vi "test Add Find Remove APU.vi"(8 "error in (no error)":errorcluster, 11 "TestCase in":refnum<class "Scripting API Test Case.lvclass">) -> (0 "error out":errorcluster, 3 "TestCase out":refnum<class "Scripting API Test Case.lvclass">)   [LabVIEW 2019, in "Scripting API Test Case.lvclass"]
uses:
  Scripting API Test Case.lvclass
  Scripting API/Custom Device/Engine Simulation Toolkit Custom Device Settings.ctl
  Scripting API/Bitfile/Bitfile.ctl
  Scripting API/APU/APU Settings.ctl
  Scripting API Test Case.lvclass/Scripting API Test Case.ctl
  <userlib>/_OpenG.lib/file/file.llb/Append Path to Root if Relative - Scalar__ogtk.vi
  <vilib>/addons/_JKI Toolkits/VI Tester/TestCase.llb/TestCase.lvclass
  Scripting API/Engine Simulation Toolkit Scripting API.lvlib
  niveristand-custom-device-testing-tools/VeriStandTestUtilities/VeriStandTestUtilities.lvlib
  C:/Program Files (x86)/National Instruments/LabVIEW 2019/vi.lib/addons/_JKI Toolkits/VI Tester/TestCase.llb/TestCase.lvclass
panel:
  in  "Save?":bool
  out "Output Filename":string
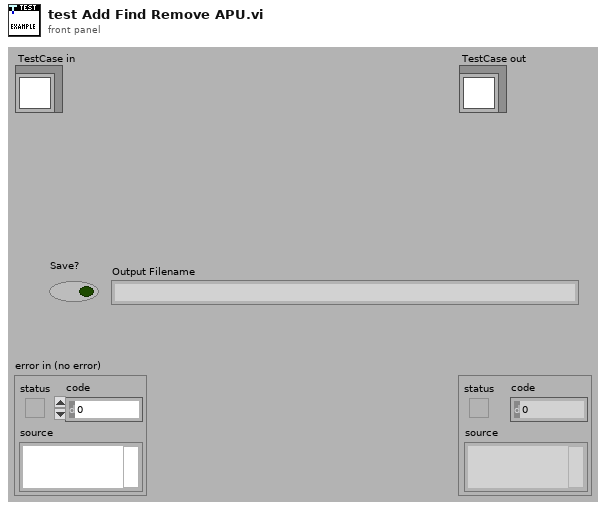
[diagram p1: front panel]
types:
  T1 = typedef "Engine Simulation Toolkit Scripting API.lvlib/APU Settings.ctl" = cluster{"Name":string, "Start angle (degrees)":dbl, "des speed":dbl, "Acceleration":bool, "des accel":dbl, "Maximum angle deviation\nbetween RIO devices (degrees)":dbl}
  T2 = typedef "Engine Simulation Toolkit Scripting API.lvlib/Bitfile.ctl" = cluster{"RIO Device Address":string, "Bitfile Path":path}
  T3 = typedef "Engine Simulation Toolkit Scripting API.lvlib/Engine Simulation Toolkit Custom Device Settings.ctl" = cluster{"Name":string, "Execution priority":enum16{"Low", "Medium", "High"}, "Rate decimation":i32, "CPU":i32}
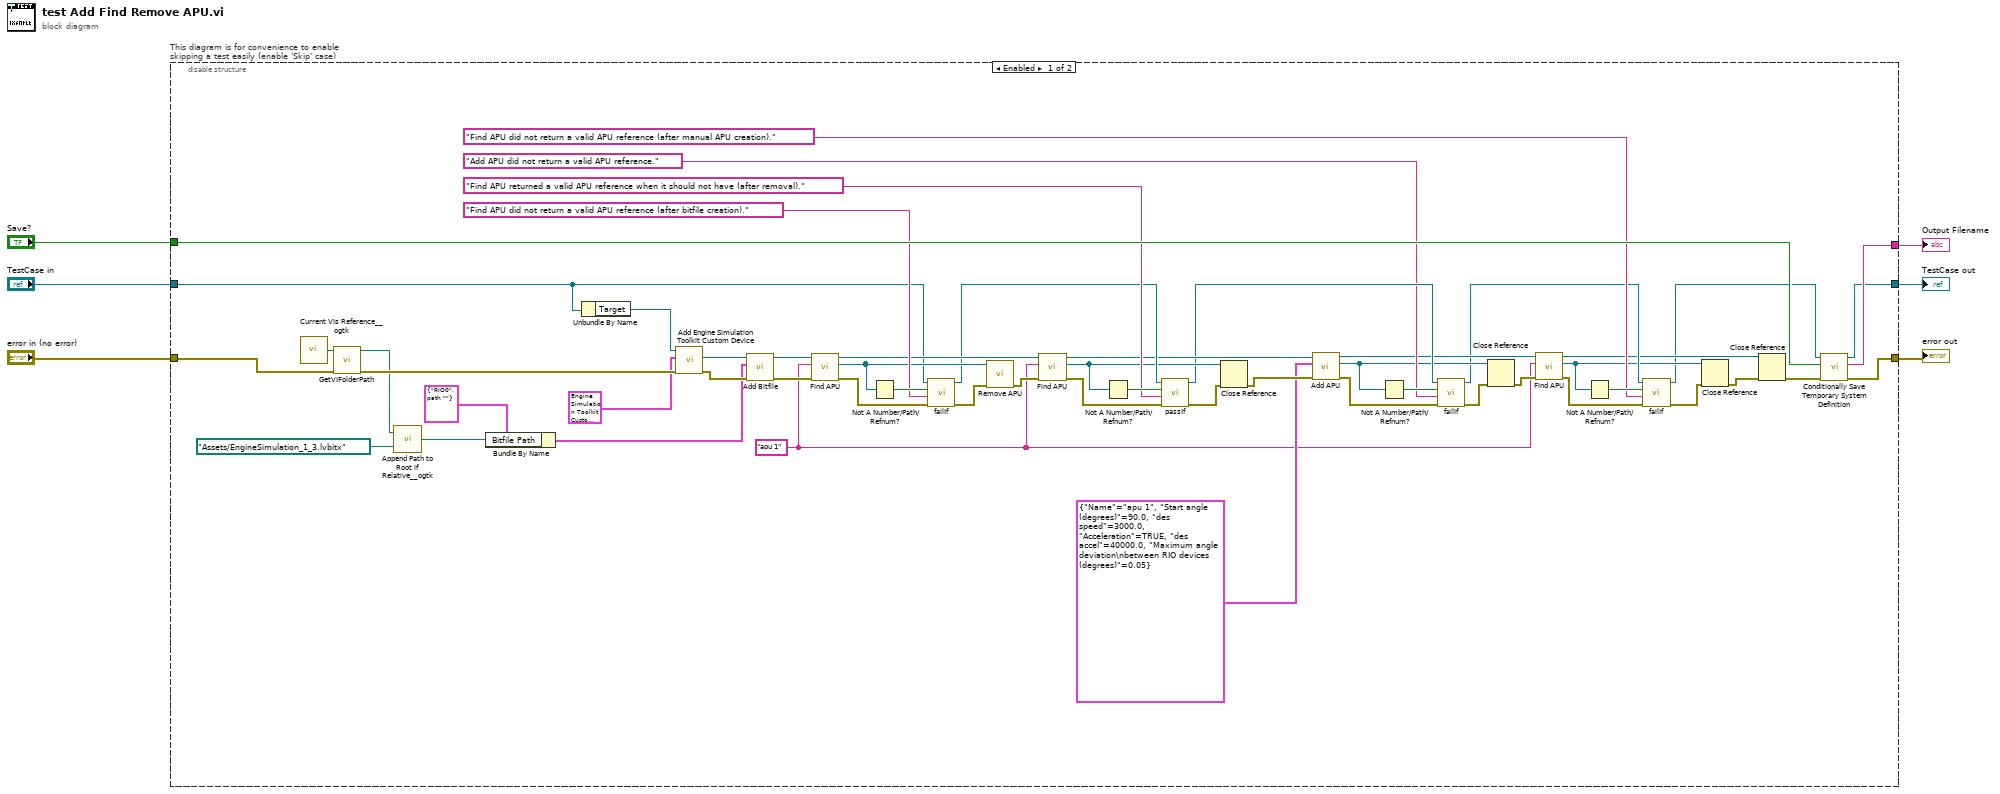
[diagram p0: block diagram]
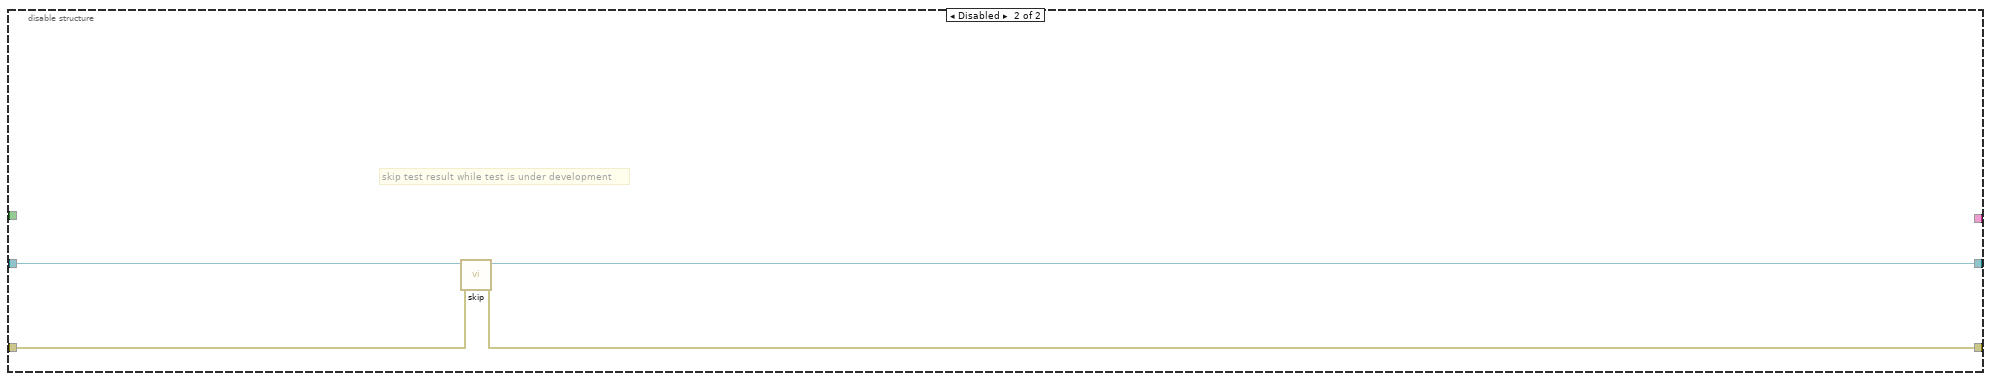
[diagram p2: hidden frame]
diagram:
  n1 = disable-structure "This diagram is for convenience to enable skipping a test easily (enable 'Skip' case)" shown="Enabled" {
    disable-tunnel: "TestCase in" -> [w10 w64]
    disable-tunnel: [w7 w62] -> w3
    disable-tunnel: [w56 w63] -> w5
    disable-tunnel: "error in (no error)" -> [w59 w61]
    disable-tunnel: [w55 _] -> w2
    disable-tunnel: "Save?" -> [w54 _]
    frame Enabled {
      w14 = "apu 1" ("Name")
      n2 = call <userlib>:"Current VIs Reference__ogtk.vi"() -> ("Current VI's reference"=w60:refnum<vi>)  [unwired: 5 in]
      n3 = call "GetVIFolderPath.vi"("error in (no error)"=w59, "VI Reference in"=w60) -> ("error out"=w58:errorcluster, "VI Folder Path out"=w50:path)  [unwired: 8 in]
      n4 = call-poly <userlib>:"Append Path to Root if Relative__ogtk.vi"("Absolute or Relative Path"=path "Assets/EngineSimulation_1_3.lvbitx", "Root Path"=w50) -> ("Absolute or Appended Path"=w46:path)
      n5 = Bundle By Name(cluster=T2 {"RIO Device Address"="RIO0", "Bitfile Path"=path ""} ("Engine Simulation Toolkit Bitfile"), "Bitfile Path"=w46) -> (w47:T2)
      n6 = Unbundle By Name(w10) -> ("Target"=w9:refnum<k24>)
      n7 = call "Add Engine Simulation Toolkit Custom Device.vi"("error in (no error)"=w58, "Settings"=T3 {"Name"="Engine Simulation Toolkit Custom Device", "Execution priority"=enum."Medium", "Rate decimation"=1, "CPU"=-2} ("Engine Simulation Toolkit Custom Device Settings"), "Target in"=w9) -> ("error out"=w51:errorcluster, "EST Custom Device"=w53:refnum<k24>)  [unwired: 6 in, 1 out]
      n8 = call "Add Bitfile.vi"("error in (no error)"=w51, "Engine Simulation Toolkit Bitfile"=w47, "EST Custom Device in"=w53) -> ("error out"=w44:errorcluster, "EST Custom Device out"=w45:refnum<k24>)  [unwired: 7 in]
      n9 = call "Find APU.vi"("error in (no error)"=w44, "Name"=w14, "EST Custom Device in"=w45) -> ("error out"=w42:errorcluster, "APU"=w39:refnum<k24>, "EST Custom Device out"=w34:refnum<k24>)  [unwired: 6 in]
      n10 = Not A Number/Path/Refnum?(number/path/refnum=w39) -> (NaN/Path/Refnum?=w43:bool)
      n11 = call-dynamic "failIf.vi"("error in (no error)"=w42, "message (\"\")"="Find APU did not return a valid APU reference (after bitfile creation)." ("message (\"\")"), "fail"=w43, "TestCase in"=w10) -> ("error out"=w40:errorcluster, "TestCase out"=w33:refnum<class "Scripting API Test Case.lvclass">)  [unwired: 6 in]
      n12 = call "Remove APU.vi"("error in (no error)"=w40, "APU"=w39) -> ("error out"=w35:errorcluster)  [unwired: 9 in]
      n13 = call "Find APU.vi"("error in (no error)"=w35, "Name"=w14, "EST Custom Device in"=w34) -> ("error out"=w37:errorcluster, "APU"=w32:refnum<k24>, "EST Custom Device out"=w30:refnum<k24>)  [unwired: 6 in]
      n14 = Not A Number/Path/Refnum?(number/path/refnum=w32) -> (NaN/Path/Refnum?=w38:bool)
      n15 = call-dynamic "passIf.vi"("error in (no error)"=w37, "message (\"\")"="Find APU returned a valid APU reference when it should not have (after removal)." ("message (\"\")"), "pass"=w38, "TestCase in"=w33) -> ("error out"=w31:errorcluster, "TestCase out"=w25:refnum<class "Scripting API Test Case.lvclass">)  [unwired: 6 in]
      n16 = Close Reference(reference=w32, error in (no error)=w31) -> (error out=w29:errorcluster)
      n17 = call "Add APU.vi"("error in (no error)"=w29, "APU Settings"=T1 {"Name"="apu 1", "Start angle (degrees)"=90.0, "des speed"=3000.0, "Acceleration"=TRUE, "des accel"=40000.0, "Maximum angle deviation\nbetween RIO devices (degrees)"=0.05}, "EST Custom Device in"=w30) -> ("error out"=w26:errorcluster, "APU"=w22:refnum<k24>, "EST Custom Device out"=w23:refnum<k24>)  [unwired: 6 in]
      n18 = Not A Number/Path/Refnum?(number/path/refnum=w22) -> (NaN/Path/Refnum?=w27:bool)
      n19 = call-dynamic "failIf.vi"("error in (no error)"=w26, "message (\"\")"="Add APU did not return a valid APU reference." ("message (\"\")"), "fail"=w27, "TestCase in"=w25) -> ("error out"=w21:errorcluster, "TestCase out"=w16:refnum<class "Scripting API Test Case.lvclass">)  [unwired: 6 in]
      n20 = Close Reference(reference=w22, error in (no error)=w21) -> (error out=w20:errorcluster)
      n21 = call "Find APU.vi"("error in (no error)"=w20, "Name"=w14, "EST Custom Device in"=w23) -> ("error out"=w17:errorcluster, "APU"=w11:refnum<k24>, "EST Custom Device out"=w15:refnum<k24>)  [unwired: 6 in]
      n22 = Not A Number/Path/Refnum?(number/path/refnum=w11) -> (NaN/Path/Refnum?=w19:bool)
      n23 = call-dynamic "failIf.vi"("error in (no error)"=w17, "message (\"\")"="Find APU did not return a valid APU reference (after manual APU creation)." ("message (\"\")"), "fail"=w19, "TestCase in"=w16) -> ("error out"=w13:errorcluster, "TestCase out"=w8:refnum<class "Scripting API Test Case.lvclass">)  [unwired: 6 in]
      n24 = Close Reference(reference=w11, error in (no error)=w13) -> (error out=w12:errorcluster)
      n25 = Close Reference(reference=w15, error in (no error)=w12) -> (error out=w57:errorcluster)
      n26 = call "Conditionally Save Temporary System Definition.vi"("error in (no error)"=w57, "Save?"=w54, "Test Case"=w8) -> ("error out"=w56:errorcluster, "filename"=w55:string, "Test Case"=w7:refnum<class "Scripting API Test Case.lvclass">)  [unwired: 6 in]
    }
    frame Disabled {
      # "skip test result while test is under development"
      n27 = call <vilib>:"skip.vi"("error in (no error)"=w61, "TestCase in"=w64) -> ("error out"=w63:errorcluster, "TestCase out"=w62:refnum<class "Scripting API Test Case.lvclass">)  [unwired: 8 in]
    }
  }
  "error out" <- w5
  "TestCase out" <- w3
  "Output Filename" <- w2
